vi "Gerador_de_Sinais.vi"() -> ()   [LabVIEW 2019]
uses:
  enum.ctl
  <vilib>/Utility/sysdir.llb/System Directory Type.ctl
  <vilib>/DAQmx/write.llb/DAQmx Write (Analog Wfm 1Chan NSamp).vi
  <vilib>/Waveform/WDTFileIO.llb/ Write Waveform to File.vi
  <vilib>/Waveform/WDTFileIO.llb/Read Waveform from File.vi
  <vilib>/Waveform/WDTOps.llb/WDT Append Waveforms DBL.vi
  <vilib>/DAQmx/create/channels.llb/DAQmx Create Channel (AO-Voltage-Basic).vi
  <vilib>/DAQmx/configure/timing.llb/DAQmx Timing (Use Waveform).vi
  <vilib>/DAQmx/miscellaneous.llb/DAQmx Fill In Error Info.vi
  <vilib>/measure/NI_MABase.lvlib
panel:
  in  "Nº de amostras":i32
  in  "Amostras/s":dbl
  in  "Canal out":tag
  in  "Input":tag
  in  "Adquirir":bool
  in  "Gerar":bool
  in  "Out mode":bool
  in  "Start":bool
  in  "conc-ops":bool
  in  "Ch2":bool
  in  "Ch1":bool
  in  "delete":bool
  in  "Escala X":dbl(knob)=0.5 min=0.5 step=0.5 scale=0.0..100.0
  in  "Conc":bool
  in  "Salvar 2":path
  in  "Salvar - opções 2":enum16{"Default", "Custom"}(ring)
  in  "Save 2":bool
  in  "Sub":bool
  in  "Add":bool
  in  "load2":bool
  in  "Carregar2":path
  out "Sinal 2":waveform(dbl)[](graph)
  in  "Salvar - opções":enum16{"Default", "Custom"}(ring)
  in  "Carregar1":path
  in  "Salvar":path
  in  "load1":bool
  in  "Save":bool
  in  "Parâmetros":T1={"Forma"=enum."Quadrada", "Amostragem"={"Amostras/s"=1000.0, "Qtde. de amostras"=1000.0}, "Frequência (Hz)"=1.0, "Amplitude (Vp)"=10.0, "Fase"=0.0, "Offset (V)"=0.0, "duty cycle (%)"=50.0} {"duty cycle (%)" format="%0.2f"; "Offset (V)" min=-10.0 max=10.0; "Fase" format="%.2p"; "Amplitude (Vp)" min=0.0 max=10.0 format="%#_13g"; "Frequência (Hz)" min=0.0 step=1.0; "Amostragem"."Qtde. de amostras" min=1000.0 step=1000.0; "Amostragem"."Amostras/s" min=0.0 format="%.2p"}
  out "Sinal":waveform(dbl)(graph)
  in  "stop":bool
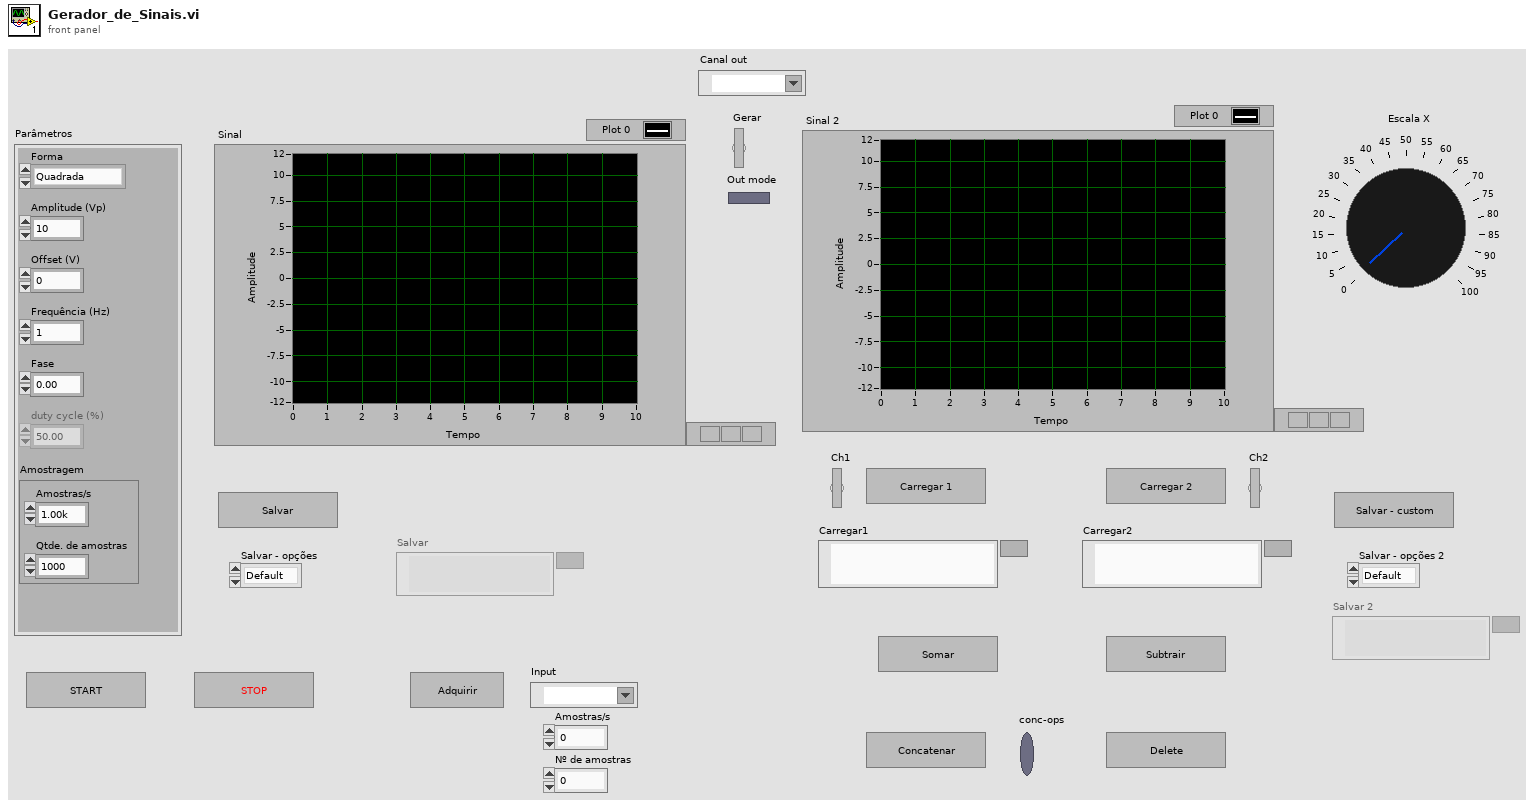
[diagram p1: front panel]
types:
  T1 = cluster{"Forma":enum16{"Quadrada", "Senoidal", "Triangular", "Dente de Serra", "Trapezoidal"}, "Amostragem":cluster{"Amostras/s":dbl, "Qtde. de amostras":dbl}, "Frequência (Hz)":dbl, "Amplitude (Vp)":dbl, "Fase":dbl, "Offset (V)":dbl, "duty cycle (%)":dbl}
  T2 = typedef "enum.ctl" = enum16{"update", "write", "stop", "save", "load1", "load2", "add", "sub", "delete", "display", "display -edit", "conc", "HW in", "HW out start", "HW out stop", "initialize", "canal out", "canal in", "save - custom"}
  T3 = cluster{"start":bool, "fila":cluster{"Operação":T2, "data":variant}}
  T4 = cluster{"onda1":waveform(dbl), "zero":waveform(dbl), "ch1":bool, "ch2":bool, "Parâmetros ":cluster{"Forma":enum16{"Quadrada", "Senoidal", "Triangular", "Dente de Serra", "Trapezoidal"}, "Amostragem":cluster{"Amostras/s":dbl, "Qtde. de amostras":dbl}, "Frequência (Hz)":dbl, "Amplitude (Vp)":dbl, "Fase":dbl, "Offset (V)":dbl, "duty cycle (%)":dbl}, "sinal":waveform(dbl), "stop ":bool, "Task out":refnum<k21>, "sinal in":waveform(dbl), "out":bool, "in":bool, "Canal in":tag, "onda 2":waveform(dbl)}
  T5 = enum8{"Enabled", "Disabled", "Disabled and Grayed Out"}
  T6 = enum16{"Quadrada", "Senoidal", "Triangular", "Dente de Serra", "Trapezoidal"}
  T7 = cluster{"Amostras/s":dbl, "Qtde. de amostras":dbl}
  T8 = typedef "System Directory Type.ctl" = i32
  T9 = typedef "LVCursorListTypeDef.ctl" = cluster{"Name":string, "Color":u32, "Style":u8, "Point Style":u8, "Name Visible":bool, "Allow Drag":bool, "Cursor Mode":u32, "Plot":i32, "Index":i32, "Position":cluster{"X":dbl, "Y":dbl}, "X Scale":u32, "Y Scale":u32, "Watch Plots":i32[], "Watch All Plots":bool, "Plot Area":i32, "Label Offset":cluster{"X":dbl, "Y":dbl}}[]
  T10 = cluster{"Name":string, "Color":u32, "Style":u8, "Point Style":u8, "Name Visible":bool, "Allow Drag":bool, "Cursor Mode":u32, "Plot":i32, "Index":i32, "Position":cluster{"X":dbl, "Y":dbl}, "X Scale":u32, "Y Scale":u32, "Watch Plots":i32[], "Watch All Plots":bool, "Plot Area":i32, "Label Offset":cluster{"X":dbl, "Y":dbl}}
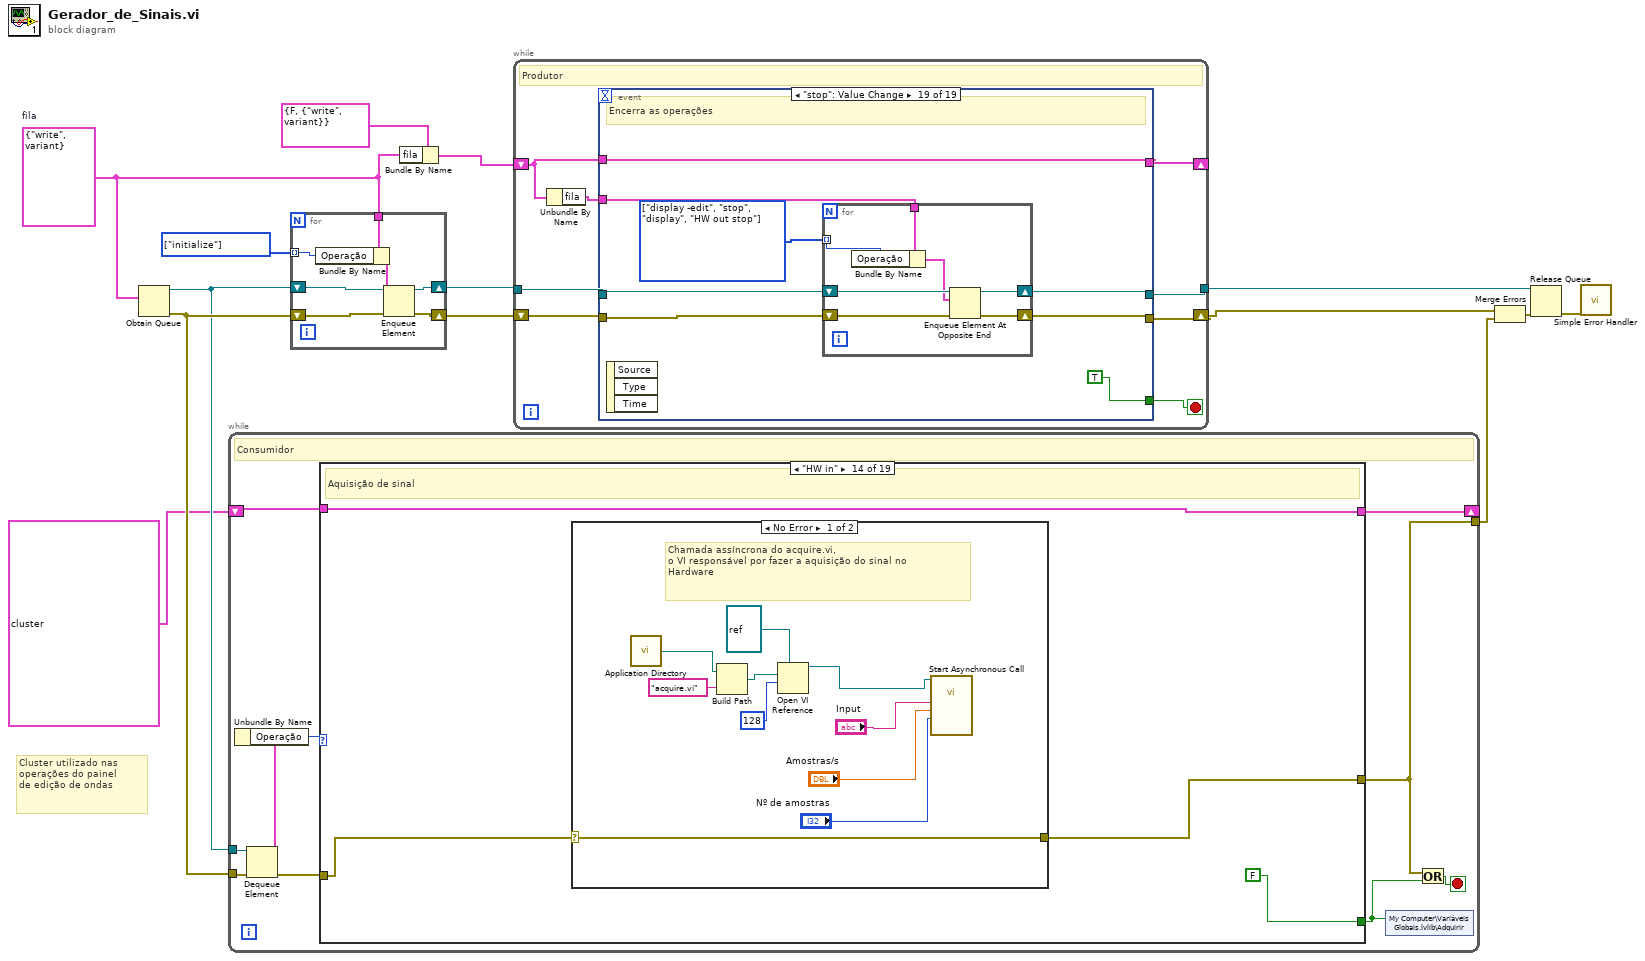
[diagram p0: block diagram]
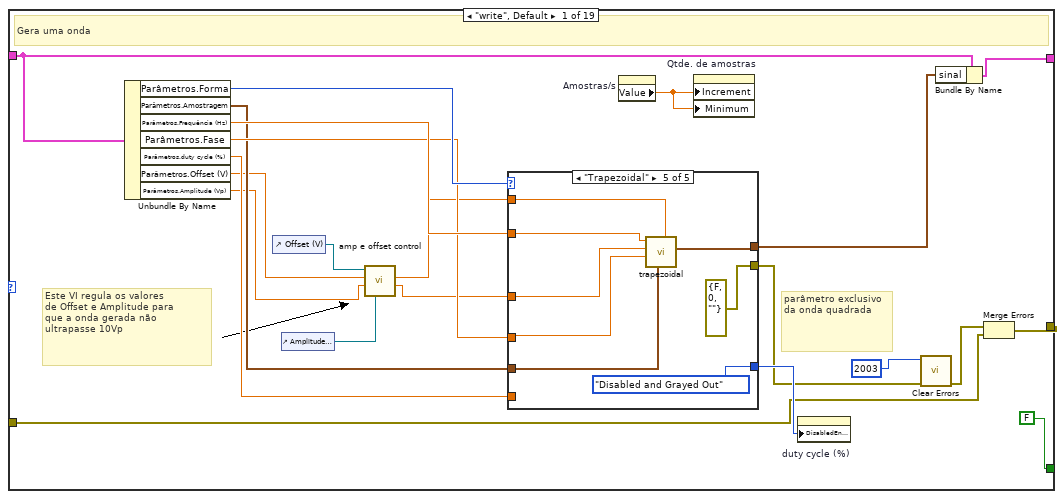
[diagram p2: hidden frame]
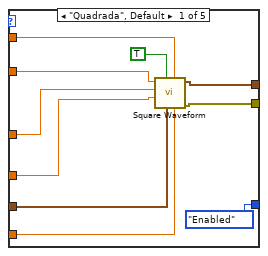
[diagram p3: hidden frame]
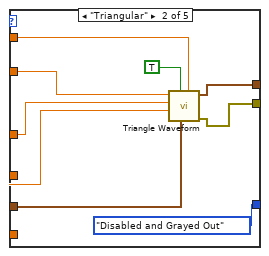
[diagram p4: hidden frame]
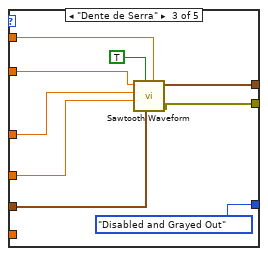
[diagram p5: hidden frame]
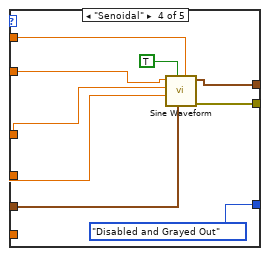
[diagram p6: hidden frame]
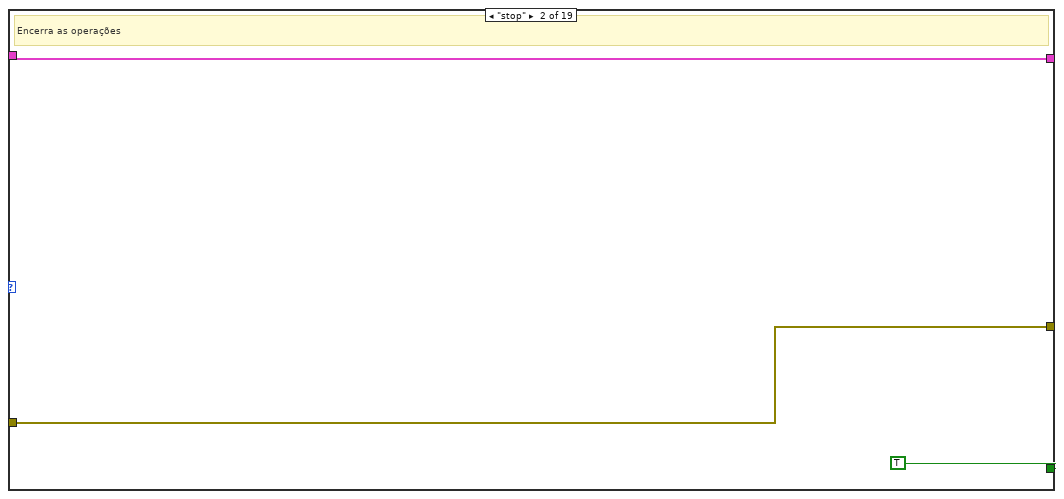
[diagram p7: hidden frame]
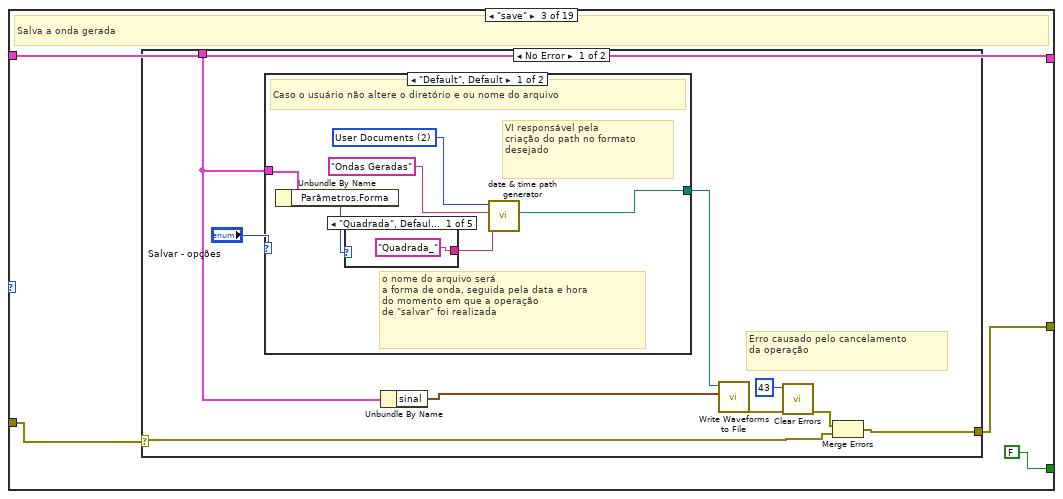
[diagram p8: hidden frame]
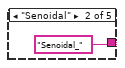
[diagram p9: hidden frame]
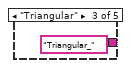
[diagram p10: hidden frame]
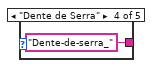
[diagram p11: hidden frame]
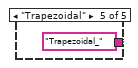
[diagram p12: hidden frame]
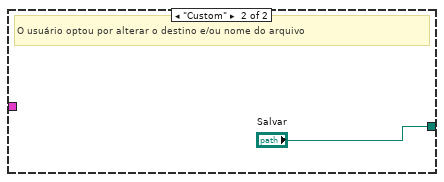
[diagram p13: hidden frame]
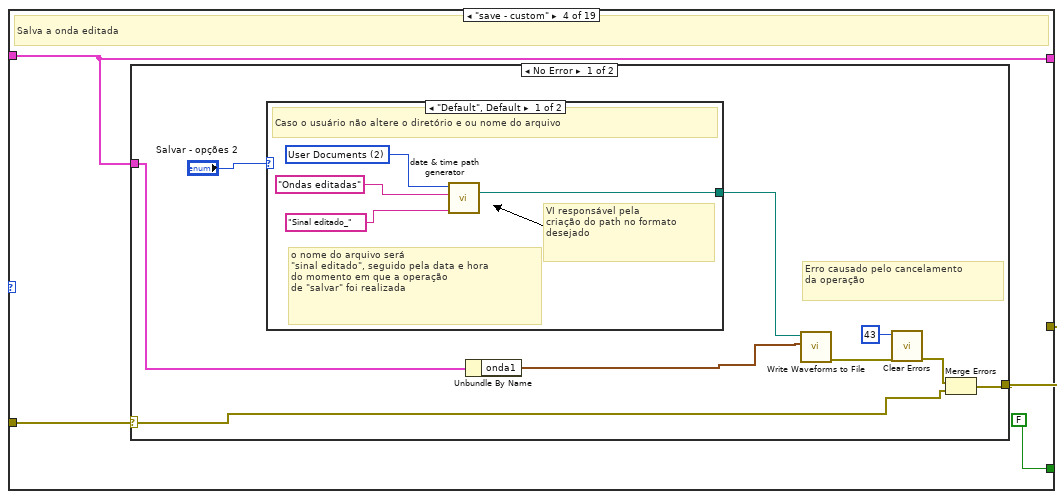
[diagram p15: hidden frame]
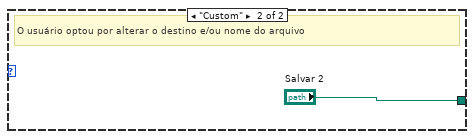
[diagram p16: hidden frame]
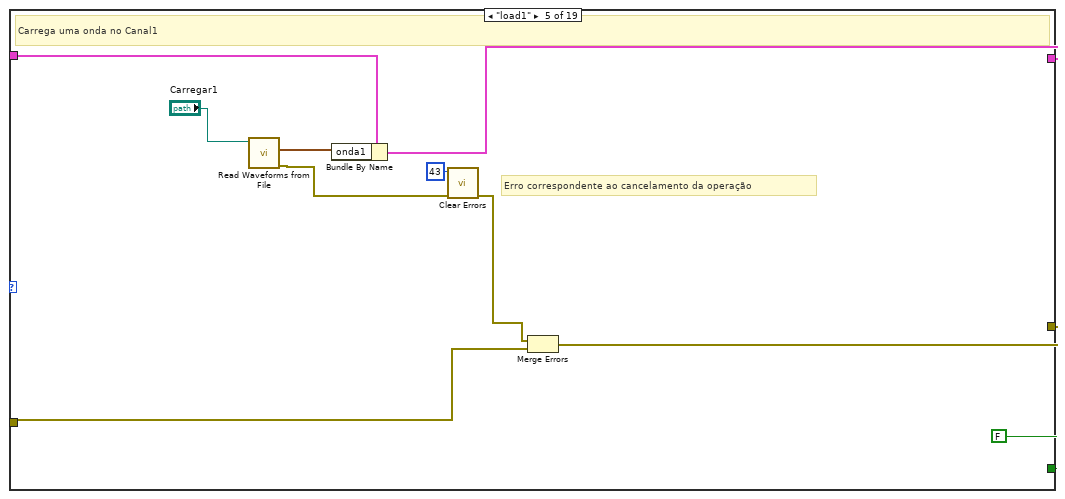
[diagram p18: hidden frame]
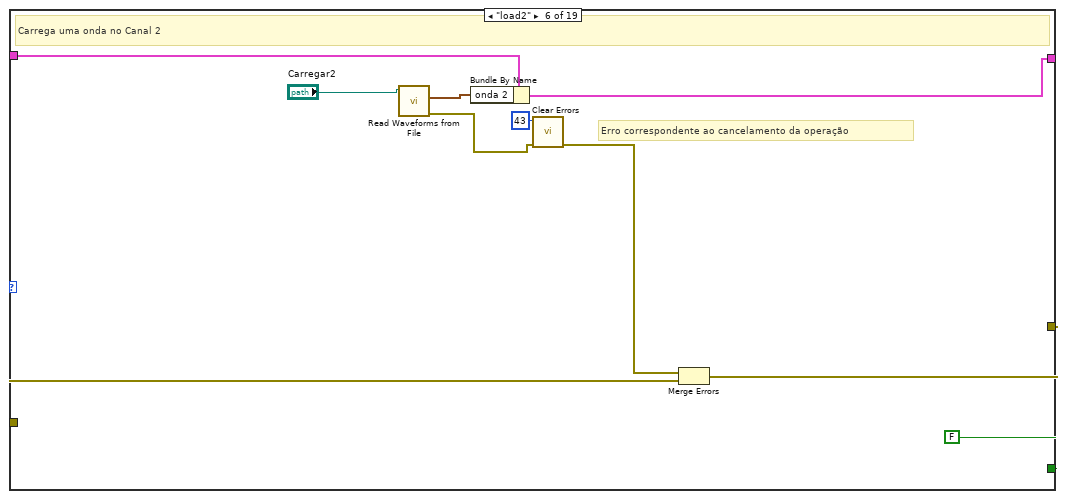
[diagram p19: hidden frame]
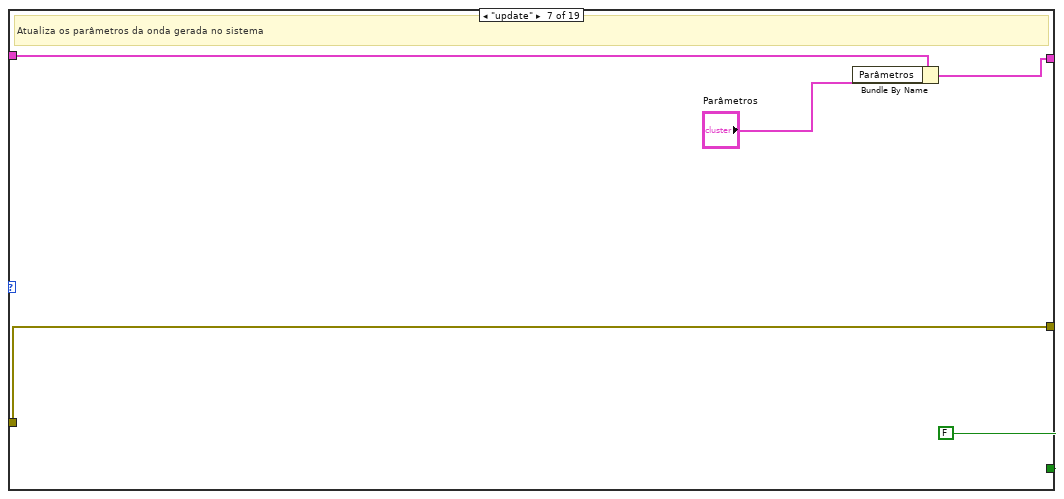
[diagram p20: hidden frame]
diagram:
  w5 = T2[] [enum."initialize"] items=["update", "write", "stop", "save", "load1", "load2", "add", "sub", "delete", "display", "display -edit", "conc", "HW in", "HW out start", "HW out stop", "initialize", "canal out", "canal in", "save - custom"]
  w4 = cluster{"Operação":T2, "data":variant} {"Operação"=enum."write", "data"=variant}  # fila
  # "Cluster utilizado nas \noperações do painel\nde edição de ondas"
  n1 = Obtain Queue(element data type=w4) -> (queue out=w11:refnum<queue>, error out=w12:errorcluster)  [unwired: 4 in, 1 out]
  n2 = while {
    shift-right: [w22] -> _
    shift-left: T4 {"onda1"={"t0"=timestamp(0 s since 1904-01-01), "dt"=1.0, "Y"=[]}, "zero"={"t0"=timestamp(0 s since 1904-01-01), "dt"=1.0, "Y"=[]}, "ch1"=TRUE, "ch2"=TRUE, "Parâmetros "={"Forma"=enum."Quadrada", "Amostragem"={"Amostras/s"=1000.0, "Qtde. de amostras"=1000.0}, "Frequência (Hz)"=1.0, "Amplitude (Vp)"=10.0, "Fase"=0.0, "Offset (V)"=0.0, "duty cycle (%)"=50.0}, "sinal"={"t0"=timestamp(0 s since 1904-01-01), "dt"=1.0, "Y"=[]}, "stop "=FALSE, "Task out"="", "sinal in"={"t0"=timestamp(0 s since 1904-01-01), "dt"=1.0, "Y"=[]}, "out"=FALSE, "in"=FALSE, "Canal in"="", "onda 2"={"t0"=timestamp(0 s since 1904-01-01), "dt"=1.0, "Y"=[]}} -> [w21]
    tunnel: w11 -> [w20]
    tunnel: w12 -> [w19]
    tunnel: [w17] -> w1
    stop <- w18 stop-if-true
    # "Consumidor"
    n3 = Dequeue Element(queue=w20, error in (no error)=w19) -> (element=w24:cluster{"Operação":T2, "data":variant}, error out=w16:errorcluster)  [unwired: 1 in, 2 out]
    n4 = Unbundle By Name(w24) -> ("Operação"=w23:T2)
    n5 = case shown="\"HW in\"" w23 {
      tunnel: [FALSE TRUE FALSE FALSE FALSE FALSE FALSE FALSE FALSE FALSE FALSE FALSE FALSE FALSE FALSE FALSE FALSE FALSE FALSE] -> w15
      tunnel: [w35 w94 w97 w123 w143 w153 w161 w173 w183 w189 w202 w226 w244 w255 w269 w302 w326 w335 w338] -> w22
      tunnel: w21 -> [w36 w94 w97 w123 w144 w154 w163 w172 w182 w188 w203 w225 w244 w255 w270 w302 w327 w336 w339]
      tunnel: w16 -> [w31 w93 w96 w121 w141 w151 w160 w165 w175 w186 w201 w223 w245 w254 w272 w300 w330 w332 w344]
      tunnel: [w33 w93 w95 w122 w140 w150 w160 w165 w175 w185 w201 w223 w245 w253 w271 w293 w329 w332 w343] -> w17
      frame "write", Default {
        # "Este VI regula os valores\nde Offset e Amplitude para\nque a onda gerada não\nultrapasse 10Vp"
        # "parâmetro exclusivo da onda quadrada"
        # "Gera uma onda"
        n6 = Unbundle By Name(w36) -> ("Parâmetros.Forma"=w43:T6, "Parâmetros.Amostragem"=w40:T7, "Parâmetros.Frequência (Hz)"=w44:dbl, "Parâmetros.Fase"=w42:dbl, "Parâmetros.duty cycle (%)"=w41:dbl, "Parâmetros.Offset (V)"=w26:dbl, "Parâmetros.Amplitude (Vp)"=w25:dbl)
        n7 = control-ref of="Offset (V)"() -> (w30:refnum<vi>)
        n8 = control-ref of="Amplitude (Vp)"() -> (w29:refnum<vi>)
        n9 = call "amp e offset control.vi"("amp ref"=w29, "Amplitude (Vp)"=w25, "Offset (V)"=w26, "offset ref"=w30) -> ("Nova Amplitude"=w28:dbl, "Novo Offset"=w27:dbl)  [unwired: 6 in]
        n10 = case shown="\"Trapezoidal\"" w43 {
          tunnel: [w56 w65 w74 w83 w90] -> w34
          tunnel: w28 -> [w55 w64 w73 w82 w91]
          tunnel: [T5."Enabled" ("Disabled") T5."Disabled and Grayed Out" ("Disabled") T5."Disabled and Grayed Out" ("Disabled") T5."Disabled and Grayed Out" ("Disabled") T5."Disabled and Grayed Out" ("Disabled")] -> w45
          tunnel: w27 -> [w51 w60 w69 w79 w87]
          tunnel: w44 -> [w52 w61 w70 w78 w88]
          tunnel: w42 -> [w50 w59 w68 w77 w86]
          tunnel: w41 -> [w49 _ _ _ _]
          tunnel: w40 -> [w48 w58 w67 w76 w85]
          tunnel: [w47 w57 w66 w75 errorcluster {"status"=FALSE, "code"=0, "source"=""} ("error out")] -> w39
          frame "Quadrada", Default {
            n11 = call <vilib>:"Square Waveform.vi"("duty cycle (%)"=w49, "offset"=w51, "sampling info"=w48, "reset signal"=TRUE, "phase"=w50, "amplitude"=w55, "frequency"=w52) -> ("error out"=w47:errorcluster, "signal out"=w56:waveform(dbl))  [unwired: 3 in]
          }
          frame "Triangular" {
            n12 = call <vilib>:"Triangle Waveform.vi"("offset"=w60, "sampling info"=w58, "reset signal"=TRUE, "phase"=w59, "amplitude"=w64, "frequency"=w61) -> ("error out"=w57:errorcluster, "signal out"=w65:waveform(dbl))  [unwired: 4 in]
          }
          frame "Dente de Serra" {
            n13 = call <vilib>:"Sawtooth Waveform.vi"("offset"=w69, "sampling info"=w67, "reset signal"=TRUE, "phase"=w68, "amplitude"=w73, "frequency"=w70) -> ("error out"=w66:errorcluster, "signal out"=w74:waveform(dbl))  [unwired: 4 in]
          }
          frame "Senoidal" {
            n14 = call <vilib>:"Sine Waveform.vi"("offset"=w79, "sampling info"=w76, "reset signal"=TRUE, "phase"=w77, "amplitude"=w82, "frequency"=w78) -> ("error out"=w75:errorcluster, "signal out"=w83:waveform(dbl))  [unwired: 4 in]
          }
          frame "Trapezoidal" {
            n15 = call "trapezoidal.vi"("offset"=w87, "sampling info"=w85, "phase"=w86, "amplitude"=w91, "frequency"=w88) -> ("signal"=w90:waveform(dbl))  [unwired: 6 in]
          }
        }
        n16 = property on="Amostras/s" class="DigNum (strict)"() -> ("Value"=w37:dbl)  [unwired: 2 in, 2 out]
        n17 = property on="Qtde. de amostras" class="DigNum (strict)"("Increment"=w37, "Minimum"=w37) -> ()  [unwired: 2 in, 2 out]
        n18 = property on="duty cycle (%)" class="DigNum (strict)"("DisabledEnum"=w45) -> ()  [unwired: 2 in, 2 out]
        n19 = call <vilib>:"Clear Errors.vi"("error in (no error)"=w39, "specific error code to clear (0: all)"=2003) -> ("error out"=w32:errorcluster)  [unwired: 4 in, 1 out]
        n20 = Bundle By Name(cluster=w36, "sinal"=w34) -> (w35:T4)
        n21 = Merge Errors(w32, w31) -> (w33:errorcluster)
      }
      frame "stop" {
        # "Encerra as operações"
      }
      frame "save" {
        # "Salva a onda gerada"
        n22 = case shown="No Error" w96 {
          selector: w96 -> [w99 w120]
          tunnel: w97 -> [w103 _]
          tunnel: [w100 w120] -> w95
          frame No Error {
            # "Erro causado pelo cancelamento\nda operação"
            n23 = case shown="\"Default\", Default" "Salvar - opções" {
              tunnel: w103 -> [w112 _]
              tunnel: [w111 "Salvar"] -> w104
              frame "Default", Default {
                w108 = T8 2 items=["User Home"=0, "User Desktop"=1, "User Documents"=2, "User Application Data"=3, "User Preferences"=4, "User Temporary"=5, "Public Documents"=6, "Public Application Data"=7, "Public Preferences"=8, "Public Cache"=13, "System Core Libraries"=9, "System Installed Libraries"=10, "Application Files"=11, "Boot Volume Root"=12] ("system directory type")
                # "VI responsável pela\ncriação do path no formato\ndesejado"
                # "o nome do arquivo será \na forma de onda, seguida pela data e hora \ndo momento em que a operação\nde \"salvar\" foi realizada"
                # "Caso o usuário não altere o diretório e ou nome do arquivo"
                n24 = Unbundle By Name(w112) -> ("Parâmetros.Forma"=w113:T6)
                n25 = case shown="\"Quadrada\", Default" w113 {
                  tunnel: ["Quadrada_" "Senoidal_" "Triangular_" "Dente-de-serra_" "Trapezoidal_"] -> w109
                  frame "Quadrada", Default {
                  }
                  frame "Senoidal" {
                  }
                  frame "Triangular" {
                  }
                  frame "Dente de Serra" {
                  }
                  frame "Trapezoidal" {
                  }
                }
                n26 = call "date & time path generator.vi"("system directory type"=w108, "nome da pasta"="Ondas Geradas" ("prompt (Create Folder)"), "nome do arquivo"=w109) -> ("path"=w111:path)  [unwired: 7 in]
              }
              frame "Custom" {
                # "O usuário optou por alterar o destino e/ou nome do arquivo"
              }
            }
            n27 = Unbundle By Name(w103) -> ("sinal"=w102:waveform(dbl))
            n28 = call-poly <vilib>:"Write Waveforms to File.vi"("waveform"=w102, "file path (dialog if empty)"=w104) -> ("error out"=w106:errorcluster)  [unwired: 8 in, 1 out]
            n29 = call <vilib>:"Clear Errors.vi"("error in (no error)"=w106, "specific error code to clear (0: all)"=43) -> ("error out"=w101:errorcluster)  [unwired: 4 in, 1 out]
            n30 = Merge Errors(w101, w99) -> (w100:errorcluster)
          }
          frame Error {
          }
        }
      }
      frame "save - custom" {
        # "Salva a onda editada"
        n31 = case shown="No Error" w121 {
          selector: w121 -> [w125 w139]
          tunnel: w123 -> [w128 _]
          tunnel: [w126 w139] -> w122
          frame No Error {
            # "Erro causado pelo cancelamento\nda operação"
            n32 = case shown="\"Default\", Default" "Salvar - opções 2" {
              tunnel: [w137 "Salvar 2"] -> w132
              frame "Default", Default {
                w136 = T8 2 items=["User Home"=0, "User Desktop"=1, "User Documents"=2, "User Application Data"=3, "User Preferences"=4, "User Temporary"=5, "Public Documents"=6, "Public Application Data"=7, "Public Preferences"=8, "Public Cache"=13, "System Core Libraries"=9, "System Installed Libraries"=10, "Application Files"=11, "Boot Volume Root"=12] ("system directory type")
                # "VI responsável pela\ncriação do path no formato\ndesejado"
                # "o nome do arquivo será \n\"sinal editado\", seguido pela data e hora \ndo momento em que a operação\nde \"salvar\" foi realizada"
                # "Caso o usuário não altere o diretório e ou nome do arquivo"
                n33 = call "date & time path generator.vi"("system directory type"=w136, "nome da pasta"="Ondas editadas" ("prompt (Create Folder)"), "nome do arquivo"="Sinal editado_") -> ("path"=w137:path)  [unwired: 7 in]
              }
              frame "Custom" {
                # "O usuário optou por alterar o destino e/ou nome do arquivo"
              }
            }
            n34 = Unbundle By Name(w128) -> ("onda1"=w131:waveform(dbl))
            n35 = call-poly <vilib>:"Write Waveforms to File.vi"("waveform"=w131, "file path (dialog if empty)"=w132) -> ("error out"=w130:errorcluster)  [unwired: 8 in, 1 out]
            n36 = call <vilib>:"Clear Errors.vi"("error in (no error)"=w130, "specific error code to clear (0: all)"=43) -> ("error out"=w127:errorcluster)  [unwired: 4 in, 1 out]
            n37 = Merge Errors(w127, w125) -> (w126:errorcluster)
          }
          frame Error {
          }
        }
      }
      frame "load1" {
        # "Erro correspondente ao cancelamento da operação"
        # "Carrega uma onda no Canal1"
        n38 = call-poly <vilib>:"Read Waveforms from File.vi"("file path (dialog if empty)"="Carregar1") -> ("error out"=w145:errorcluster, "first waveform in record"=w147:waveform(dbl))  [unwired: 5 in, 2 out]
        n39 = Bundle By Name(cluster=w144, "onda1"=w147) -> (w143:T4)
        n40 = call <vilib>:"Clear Errors.vi"("error in (no error)"=w145, "specific error code to clear (0: all)"=43) -> ("error out"=w142:errorcluster)  [unwired: 4 in, 1 out]
        n41 = Merge Errors(w142, w141) -> (w140:errorcluster)
      }
      frame "load2" {
        # "Erro correspondente ao cancelamento da operação"
        # "Carrega uma onda no Canal 2"
        n42 = call-poly <vilib>:"Read Waveforms from File.vi"("file path (dialog if empty)"="Carregar2") -> ("error out"=w156:errorcluster, "first waveform in record"=w157:waveform(dbl))  [unwired: 5 in, 2 out]
        n43 = Bundle By Name(cluster=w154, "onda 2"=w157) -> (w153:T4)
        n44 = call <vilib>:"Clear Errors.vi"("error in (no error)"=w156, "specific error code to clear (0: all)"=43) -> ("error out"=w152:errorcluster)  [unwired: 4 in, 1 out]
        n45 = Merge Errors(w152, w151) -> (w150:errorcluster)
      }
      frame "update" {
        # "Atualiza os parâmetros da onda gerada no sistema"
        n46 = Bundle By Name(cluster=w163, "Parâmetros"="Parâmetros") -> (w161:T4)
      }
      frame "add" {
        # "o sinal resultante substitui aquele carregado no canal1"
        # "adição dos sinais do canal 1 e do \ncanal2 e normalização do sinal resultante \ndentro do limite estabelicdo"
        # "Adição de 2 ondas"
        n47 = Unbundle By Name(w172) -> ("onda1"=w167:waveform(dbl), "onda 2"=w166:waveform(dbl))
        n48 = call "add or sub waveforms.vi"("operation"=TRUE, "inf"=-10.0, "Waveform 2"=w166, "Waveform 1"=w167, "sup"=10.0) -> ("New Waveform"=w168:waveform(dbl))  [unwired: 6 in]
        n49 = Bundle By Name(cluster=w172, "onda1"=w168) -> (w173:T4)
      }
      frame "sub" {
        # "subtração dos sinais do canal 1 e do \ncanal2 e normalização do sinal resultante \ndentro do limite estabelicdo"
        # "o sinal resultante substitui aquele carregado no canal1"
        # "Subtração de 2 ondas"
        n50 = Unbundle By Name(w182) -> ("onda1"=w181:waveform(dbl), "onda 2"=w180:waveform(dbl))
        n51 = call "add or sub waveforms.vi"("operation"=FALSE, "inf"=-10.0, "Waveform 2"=w180, "Waveform 1"=w181, "sup"=10.0) -> ("New Waveform"=w179:waveform(dbl))  [unwired: 6 in]
        n52 = Bundle By Name(cluster=w182, "onda1"=w179) -> (w183:T4)
      }
      frame "conc" {
        # "Concatenar 2 ondas"
        n53 = Unbundle By Name(w188) -> ("onda1"=w194:waveform(dbl), "onda 2"=w192:waveform(dbl))
        n54 = case shown="True" "conc-ops" {
          tunnel: [w198 w199] -> w193
          tunnel: w194 -> [w198 w200]
          tunnel: w192 -> [w197 w199]
          tunnel: [w197 w200] -> w191
          frame False {
            # "A onda2 começa depois da1"
          }
          frame True {
            # "A onda 2 começa antes da 1"
          }
        }
        n55 = call-poly <vilib>:"Append Waveforms.vi"("waveform B"=w191, "waveform A"=w193) -> ("error out"=w187:errorcluster, "waveform out"=w195:waveform(dbl))  [unwired: 8 in]
        n56 = Bundle By Name(cluster=w188, "onda1"=w195) -> (w189:T4)
        n57 = Merge Errors(w187, w186) -> (w185:errorcluster)
      }
      frame "delete" {
        # "Deleta o trecho \"entre cursores\"da onda apresentada no display"
        n58 = Unbundle By Name(w203) -> ("ch1"=w204:bool, "ch2"=w205:bool)
        n59 = Or(x=w204, y=w205) -> (x .or. y?=w206:bool)
        n60 = case shown="True" w206 {
          tunnel: w203 -> [w208 w213]
          tunnel: [w208 w216] -> w202
          tunnel: w204 -> [_ w212]
          frame False {
            # "Se os dois canais estiverem desabilitados, nada acontece"
          }
          frame True {
            # "Se o canal1 estiver\nativo, sua onda será editada.\nCaso o contrário, a onda do canal2 será \neditada"
            # "Pelo menos um canal está ativo"
            n61 = Unbundle By Name(w213) -> ("onda1"=w215:waveform(dbl), "onda 2"=w214:waveform(dbl))
            n62 = Select(t=w215, s=w212, f=w214) -> (s? t:f=w211:waveform(dbl))
            n63 = control-ref of="Sinal 2"() -> (w209:refnum<vi>)
            n64 = call "deleta trecho de onda.vi"("Waveform"=w211, "reference"=w209) -> ("New Waveform"=w210:waveform(dbl))  [unwired: 9 in]
            n65 = case shown="True" w212 {
              tunnel: w210 -> [w219 w222]
              tunnel: [w217 w221] -> w216
              tunnel: w213 -> [w218 w220]
              frame False {
                # "A onda 2 foi editada"
                n66 = Bundle By Name(cluster=w218, "onda 2"=w219) -> (w217:T4)
              }
              frame True {
                # "A onda1 foi editada"
                n67 = Bundle By Name(cluster=w220, "onda1"=w222) -> (w221:T4)
              }
            }
          }
        }
      }
      frame "display -edit" {
        # "Atualiza o display de edição"
        n68 = Bundle By Name(cluster=w225, "ch2"="Ch2", "ch1"="Ch1", "stop"="stop") -> (w230:T4)
        n69 = case shown="True" "stop" {
          tunnel: w230 -> [w240 w243]
          tunnel: [w240 w243] -> w226
          tunnel: "Ch1" -> [w239 _]
          tunnel: "Ch2" -> [w237 _]
          tunnel: [w238 w242] -> w227
          frame False {
            # "canal 1"
            # "canal 2"
            # "Stop não foi pressionado"
            n70 = Unbundle By Name(w240) -> ("onda 2"=w235:waveform(dbl), "zero"=w234:waveform(dbl), "onda1"=w236:waveform(dbl))
            n71 = Select(t=w235, s=w237, f=w234) -> (s? t:f=w232:waveform(dbl))
            n72 = Select(t=w236, s=w239, f=w234) -> (s? t:f=w233:waveform(dbl))
            n73 = Build Array(w233, w232) -> (w238:waveform(dbl)[])
          }
          frame True {
            # "Limpa o display"
            # "Stop foi pressionado"
            n74 = Unbundle By Name(w243) -> ("zero"=w241:waveform(dbl))
            n75 = Build Array(w241, w241) -> (w242:waveform(dbl)[])
          }
        }
        "Sinal 2" <- w227
      }
      frame "display" {
        n76 = Unbundle By Name(w244) -> ("stop"=w248:bool)
        n77 = case shown="True" w248 {
          tunnel: w244 -> [w250 w252]
          tunnel: [w249 w251] -> w247
          frame False {
            n78 = Unbundle By Name(w250) -> ("sinal"=w249:waveform(dbl))
          }
          frame True {
            n79 = Unbundle By Name(w252) -> ("zero"=w251:waveform(dbl))
          }
        }
        "Sinal" <- w247
      }
      frame "HW in" {
        # "Aquisição de sinal"
        n80 = case shown="No Error" w254 {
          selector: w254 -> [w257 w267]
          tunnel: [w257 w267] -> w253
          frame No Error {
            # "Chamada assíncrona do acquire.vi,\no VI responsável por fazer a aquisição do sinal no\nHardware"
            n81 = call <vilib>:"Application Directory.vi"() -> ("Application Directory"=w266:path)
            n82 = Build Path(base path=w266, name or relative path="acquire.vi") -> (appended path=w264:path)
            n83 = Open VI Reference(type specifier VI Refnum (for type only)=refnum<vi> refnum, vi path=w264, options=128) -> (vi reference=w262:refnum<vi>)  [unwired: 3 in, 1 out]
            n84 = call-by-ref "Start Asynchronous Call"(reference=w262, "Number of Samples"="Nº de amostras", "Sample Rate"="Amostras/s", "Physical Channel"="Input") -> ()  [unwired: 9 in, 3 out]
          }
          frame Error {
          }
        }
      }
      frame "HW out start" {
        # "Gerar forma de onda no HW"
        n85 = case shown="No Error" w272 {
          selector: w272 -> [w289 w291]
          tunnel: w270 -> [w274 w292]
          tunnel: [w287 w291] -> w271
          tunnel: [w290 w292] -> w269
          frame No Error {
            w283 = 10123 items=["Finite Samples"=10178, "Continuous Samples"=10123, "Hardware Timed Single Point"=12522] ("sample mode")
            # "Flag \"out\" será utilizada \nno estado HW out stop, \npara que o programa verifique\nse é necessário finalizar a task antes\nde encerrar o VI"
            # "seleciona a onda a ser\ngerada no HW."
            n86 = Unbundle By Name(w274) -> ("onda1"=w285:waveform(dbl), "sinal"=w284:waveform(dbl))
            n87 = call-poly <vilib>:"DAQmx Create Virtual Channel.vi"("physical channels"="Canal out", "error in"=w289) -> ("task out"=w276:refnum<k21>, "error out"=w277:errorcluster)  [unwired: 12 in]
            n88 = Select(t=w285, s="Out mode", f=w284) -> (s? t:f=w282:waveform(dbl))
            n89 = call-poly <vilib>:"DAQmx Timing.vi"("task/channels in"=w276, "sample mode"=w283, "waveform"=w282, "error in"=w277) -> ("task out"=w281:refnum<k21>, "error out"=w280:errorcluster)  [unwired: 10 in]
            n90 = call-poly <vilib>:"DAQmx Write.vi"("task/channels in"=w281, "data"=w282, "error in"=w280) -> ("task out"=w279:refnum<k21>, "error out"=w278:errorcluster)  [unwired: 10 in, 1 out]
            n91 = call <vilib>:"DAQmx Start Task.vi"("task/channels in"=w279, "error in"=w278) -> ("task out"=w288:refnum<k21>, "error out"=w287:errorcluster)  [unwired: 12 in]
            n92 = Bundle By Name(cluster=w274, "Task out"=w288, "out"=TRUE) -> (w290:T4)
          }
          frame Error {
          }
        }
      }
      frame "initialize" {
        w296 = T5."Enabled" ("Disabled")
        w303 = 1000.0 ("Value")
        # "Inicialização do programa"
        n93 = property on="Sinal 2" class="WFGraph (strict)"(error in=w300) -> (error out=w299:errorcluster, "CrsrList"=w317:T9)  [unwired: 1 in, 1 out]
        n94 = Index Array(array=w317, index=1) -> (element=w316:T10)
        n95 = Index Array(array=w317, index=0) -> (element=w315:T10)
        n96 = Bundle By Name(cluster=w316, "Position.Y"=0.0) -> (w319:T10)
        n97 = property on="Adquirir" class="Bool"(error in=w299, "DisabledEnum"=w296) -> (error out=w298:errorcluster)  [unwired: 1 in, 1 out]
        n98 = Bundle By Name(cluster=w315, "Position.Y"=0.0) -> (w318:T10)
        n99 = property on="Gerar" class="Bool (strict)"(error in=w298, "DisabledEnum"=w296) -> (error out=w297:errorcluster)  [unwired: 1 in, 1 out]
        n100 = Replace Array Subset(array=w317, new element=w318, index=0) -> (w320:T9)
        n101 = Replace Array Subset(array=w320, new element=w319, index=1) -> (w321:T9)
        n102 = property on="Sinal 2" class="WFGraph (strict)"(error in=w297, "CrsrList"=w321) -> (error out=w322:errorcluster)  [unwired: 1 in, 1 out]
        n103 = property on="Salvar - opções" class="Enum (strict)"(error in=w322, "Value"=enum16{"Default", "Custom"}."Default" ("Salvar - opções")) -> (error out=w314:errorcluster)  [unwired: 1 in, 1 out]
        n104 = property on="Salvar" class="Path"(error in=w314, "DisabledEnum"=T5."Disabled and Grayed Out" ("Disabled")) -> (error out=w312:errorcluster)  [unwired: 1 in, 1 out]
        n105 = property on="Amostras/s" class="DigNum (strict)"(error in=w312, "Value"=w303) -> (error out=w313:errorcluster)  [unwired: 1 in, 1 out]
        n106 = property on="Qtde. de amostras" class="DigNum (strict)"(error in=w313, "Value"=w303) -> (error out=w295:errorcluster)  [unwired: 1 in, 1 out]
        n107 = property on="Gerar" class="Bool (strict)"(error in=w295, "Value"=FALSE ("Gerar")) -> (error out=w293:errorcluster)  [unwired: 1 in, 1 out]
      }
      frame "canal out" {
        # "Seleção do canal de saída"
        n108 = property on="Gerar" class="Bool (strict)"("DisabledEnum"=T5."Enabled" ("Disabled")) -> ()  [unwired: 2 in, 2 out]
        n109 = call-poly <vilib>:"DAQmx Create Virtual Channel.vi"("physical channels"=tag "Dev1/ao0", "error in"=w330) -> ("task out"=w328:refnum<k21>, "error out"=w329:errorcluster)  [unwired: 12 in]
        n110 = Bundle By Name(cluster=w327, "Task out"=w328) -> (w326:T4)
      }
      frame "canal in" {
        w331 = tag ""  # Canal in
        n111 = property on="Adquirir" class="Bool"("DisabledEnum"=T5."Enabled" ("Disabled")) -> ()  [unwired: 2 in, 2 out]
        n112 = Bundle By Name(cluster=w336, "Canal in"=w331) -> (w335:T4)
      }
      frame "HW out stop" {
        # "A flag \"out\" indica se\né necessário interromper a task ao\nchegar neste estado"
        # "Finaliza a task do output do HW"
        n113 = Unbundle By Name(w339) -> ("out"=w340:bool, "Task out"=w341:refnum<k21>)
        n114 = case shown="False" w340 {
          tunnel: w344 -> [w345 w350]
          tunnel: [w345 w347] -> w343
          tunnel: w341 -> [_ w348]
          frame False {
          }
          frame True {
            n115 = call <vilib>:"DAQmx Stop Task.vi"("task/channels in"=w348, "error in"=w350) -> ("task out"=w346:refnum<k21>, "error out"=w349:errorcluster)  [unwired: 12 in]
            n116 = call <vilib>:"DAQmx Clear Task.vi"("task in"=w346, "error in"=w349) -> ("error out"=w347:errorcluster)  [unwired: 13 in]
          }
        }
        n117 = Bundle By Name(cluster=w339, "out"=FALSE) -> (w338:T4)
      }
    }
    n118 = shared-variable "My Computer\\Variáveis Globais.lvlib\\Adquirir"(w15) -> ()  [unwired: 1 in, 1 out]
    n119 = Or(x=w17, y=w15) -> (x .or. y?=w18:bool)
  }
  n120 = for {
    tunnel: w4 -> [w352]
    shift-right: [w353] -> w8
    shift-left: w12 -> [w357]
    shift-right: [w354] -> w9
    shift-left: w11 -> [w356]
    tunnel: w5 -> [w351] mode=indexing
    n121 = Bundle By Name(cluster=w352, "Operação"=w351) -> (w355:cluster{"Operação":T2, "data":variant})
    n122 = Enqueue Element(queue=w356, element=w355, error in (no error)=w357) -> (queue out=w354:refnum<queue>, error out=w353:errorcluster)  [unwired: 1 in, 1 out]
  }
  n123 = Bundle By Name(cluster=T3 {"start"=FALSE, "fila"={"Operação"=enum."write", "data"=variant}}, "fila"=w4) -> (w7:T3)
  n124 = while {
    shift-right: [w363] -> w2
    shift-left: w8 -> [w361]
    tunnel: w9 -> [w362]
    tunnel: [w364] -> w14
    shift-right: [w358] -> _
    shift-left: w7 -> [w360]
    stop <- w365 stop-if-true
    # "Produtor"
    n125 = Unbundle By Name(w360) -> ("fila"=w359:cluster{"Operação":T2, "data":variant})
    n126 = event shown="[18] \"stop\": Value Change" {
      selector: _ -> [_ _ _ _ _ _ _ _ _ _ _ _ _ _ _ _ _ _ _]
      dyn-events: _ -> [_ _ _ _ _ _ _ _ _ _ _ _ _ _ _ _ _ _ _]
      timeout: _ -> [_ _ _ _ _ _ _ _ _ _ _ _ _ _ _ _ _ _ _]
      tunnel: w362 -> [w372 w397 w409 w418 w432 w449 w461 w476 w491 w509 w520 w527 w542 w557 w569 w578 w587 w596 w606]
      tunnel: w361 -> [w371 w396 w410 w419 w430 w446 w462 w477 w492 w510 w518 w528 w543 w558 w568 w577 w586 w595 w605]
      tunnel: [FALSE FALSE FALSE FALSE FALSE FALSE FALSE FALSE FALSE FALSE FALSE FALSE FALSE FALSE FALSE FALSE FALSE FALSE TRUE] -> w365
      tunnel: [w370 w394 w411 w420 w427 w441 w459 w474 w489 w511 w517 w525 w540 w555 w568 w579 w588 w597 w603] -> w363
      tunnel: [w369 w395 w412 w421 w431 w448 w460 w475 w490 w512 w516 w526 w541 w556 w569 w580 w589 w598 w604] -> w364
      tunnel: [w367 w391 w407 w416 w424 w440 w458 w473 w488 w506 w519 w524 w539 w554 w567 w574 w583 w592 w602] -> w358
      tunnel: w360 -> [w367 w392 w407 w416 w424 w440 w458 w473 w488 w506 w519 w524 w539 w554 w567 w574 w583 w592 w602]
      tunnel: w359 -> [w366 w390 w406 w415 _ _ w457 w472 w487 w505 w515 w523 w538 w553 _ w573 w582 w591 w601]
      event "Parâmetros": Value Change {
        # "Se houver uma alteração em qualquer parâmetro do sinal, uma nova Waveform é gerada"
        n127 = event-data() -> ()  [unwired: 1 in, 3 out]
        n128 = Unbundle By Name(w367) -> ("start"=w368:bool)
        n129 = case shown="True" w368 {
          tunnel: w372 -> [w375 w381]
          tunnel: w371 -> [w374 w380]
          tunnel: [w374 w378] -> w370
          tunnel: [w375 w379] -> w369
          tunnel: w366 -> [_ w377]
          frame False {
          }
          frame True {
            w376 = T2[] [enum."update", enum."write", enum."display"] items=["update", "write", "stop", "save", "load1", "load2", "add", "sub", "delete", "display", "display -edit", "conc", "HW in", "HW out start", "HW out stop", "initialize", "canal out", "canal in", "save - custom"]
            n130 = for {
              tunnel: w377 -> [w384]
              tunnel: w376 -> [w382] mode=indexing
              shift-right: [w386] -> w379
              shift-left: w381 -> [w388]
              shift-right: [w385] -> w378
              shift-left: w380 -> [w387]
              n131 = Bundle By Name(cluster=w384, "Operação"=w382) -> (w383:cluster{"Operação":T2, "data":variant})
              n132 = Enqueue Element(queue=w388, element=w383, error in (no error)=w387) -> (queue out=w386:refnum<queue>, error out=w385:errorcluster)  [unwired: 1 in, 1 out]
            }
          }
        }
      }
      event "Start": Value Change {
        w389 = T2[] [enum."update", enum."write", enum."display"] items=["update", "write", "stop", "save", "load1", "load2", "add", "sub", "delete", "display", "display -edit", "conc", "HW in", "HW out start", "HW out stop", "initialize", "canal out", "canal in", "save - custom"]
        # "Se houver uma alteração em qualquer parâmetro do sinal, uma nova Waveform é gerada"
        n133 = event-data() -> ()  [unwired: 1 in, 5 out]
        n134 = for {
          tunnel: w389 -> [w399] mode=indexing
          tunnel: w390 -> [w400]
          shift-right: [w403] -> w395
          shift-left: w397 -> [w405]
          shift-right: [w402] -> w394
          shift-left: w396 -> [w404]
          n135 = Bundle By Name(cluster=w400, "Operação"=w399) -> (w401:cluster{"Operação":T2, "data":variant})
          n136 = Enqueue Element(queue=w405, element=w401, error in (no error)=w404) -> (queue out=w403:refnum<queue>, error out=w402:errorcluster)  [unwired: 1 in, 1 out]
        }
        n137 = Bundle By Name(cluster=w392, "start"="Start") -> (w391:T3)
      }
      event "Save": Value Change {
        # "Salvar a onda gerada"
        n138 = event-data() -> ()  [unwired: 1 in, 5 out]
        n139 = Bundle By Name(cluster=w406, "Operação"=enum."save") -> (w408:cluster{"Operação":T2, "data":variant})
        n140 = Enqueue Element(queue=w409, element=w408, error in (no error)=w410) -> (queue out=w412:refnum<queue>, error out=w411:errorcluster)  [unwired: 1 in, 1 out]
      }
      event "Save 2": Value Change {
        # "Salvar a onda editada"
        n141 = event-data() -> ()  [unwired: 1 in, 5 out]
        n142 = Bundle By Name(cluster=w415, "Operação"=enum."save - custom") -> (w417:cluster{"Operação":T2, "data":variant})
        n143 = Enqueue Element(queue=w418, element=w417, error in (no error)=w419) -> (queue out=w421:refnum<queue>, error out=w420:errorcluster)  [unwired: 1 in, 1 out]
      }
      event "Salvar - opções": Value Change {
        # "Habilita/desabilita as formas de \"salvar\""
        n144 = event-data() -> ()  [unwired: 1 in, 5 out]
        n145 = property on="Salvar - opções" class="Enum (strict)"(error in=w430) -> (error out=w429:errorcluster, "Value"=w433:enum16{"Default", "Custom"})  [unwired: 1 in, 1 out]
        n146 = case shown="\"Default\", Default" w433 {
          tunnel: w432 -> [w436 w439]
          tunnel: [w436 w439] -> w431
          tunnel: w429 -> [w434 w438]
          tunnel: [w434 w438] -> w426
          tunnel: [T5."Disabled and Grayed Out" ("Disabled") T5."Enabled" ("Disabled")] -> w425
          frame "Default", Default {
          }
          frame "Custom" {
          }
        }
        n147 = property on="Salvar" class="Path"(error in=w426, "DisabledEnum"=w425) -> (error out=w427:errorcluster)  [unwired: 1 in, 1 out]
      }
      event "Salvar - opções 2": Value Change {
        # "Habilita/desabilita as formas de \"salvar\""
        n148 = event-data() -> ()  [unwired: 1 in, 5 out]
        n149 = property on="Salvar - opções 2" class="Enum (strict)"(error in=w446) -> (error out=w445:errorcluster, "Value"=w444:enum16{"Default", "Custom"})  [unwired: 1 in, 1 out]
        n150 = case shown="\"Default\", Default" w444 {
          tunnel: w449 -> [w452 w455]
          tunnel: [w452 w455] -> w448
          tunnel: w445 -> [w450 w454]
          tunnel: [w450 w454] -> w442
          tunnel: [T5."Disabled and Grayed Out" ("Disabled") T5."Enabled" ("Disabled")] -> w443
          frame "Default", Default {
          }
          frame "Custom" {
          }
        }
        n151 = property on="Salvar 2" class="Path"(error in=w442, "DisabledEnum"=w443) -> (error out=w441:errorcluster)  [unwired: 1 in, 1 out]
      }
      event "load1": Value Change {
        w456 = T2[] [enum."load1", enum."display -edit"] items=["update", "write", "stop", "save", "load1", "load2", "add", "sub", "delete", "display", "display -edit", "conc", "HW in", "HW out start", "HW out stop", "initialize", "canal out", "canal in", "save - custom"]
        # "Carrega uma onda para o canal 1"
        n152 = event-data() -> ()  [unwired: 1 in, 5 out]
        n153 = for {
          tunnel: w456 -> [w468] mode=indexing
          tunnel: w457 -> [w464]
          shift-right: [w466] -> w459
          shift-left: w462 -> [w470]
          shift-right: [w467] -> w460
          shift-left: w461 -> [w469]
          n154 = Bundle By Name(cluster=w464, "Operação"=w468) -> (w465:cluster{"Operação":T2, "data":variant})
          n155 = Enqueue Element(queue=w469, element=w465, error in (no error)=w470) -> (queue out=w467:refnum<queue>, error out=w466:errorcluster)  [unwired: 1 in, 1 out]
        }
      }
      event "load2": Value Change {
        w471 = T2[] [enum."load2", enum."display -edit"] items=["update", "write", "stop", "save", "load1", "load2", "add", "sub", "delete", "display", "display -edit", "conc", "HW in", "HW out start", "HW out stop", "initialize", "canal out", "canal in", "save - custom"]
        # "Carrega uma onda para o canal 2"
        n156 = event-data() -> ()  [unwired: 1 in, 5 out]
        n157 = for {
          tunnel: w472 -> [w480]
          shift-right: [w482] -> w474
          shift-left: w477 -> [w485]
          shift-right: [w483] -> w475
          shift-left: w476 -> [w484]
          tunnel: w471 -> [w479] mode=indexing
          n158 = Bundle By Name(cluster=w480, "Operação"=w479) -> (w481:cluster{"Operação":T2, "data":variant})
          n159 = Enqueue Element(queue=w484, element=w481, error in (no error)=w485) -> (queue out=w483:refnum<queue>, error out=w482:errorcluster)  [unwired: 1 in, 1 out]
        }
      }
      event "Add": Value Change {
        w486 = T2[] [enum."add", enum."display -edit"] items=["update", "write", "stop", "save", "load1", "load2", "add", "sub", "delete", "display", "display -edit", "conc", "HW in", "HW out start", "HW out stop", "initialize", "canal out", "canal in", "save - custom"]
        # "Adição"
        n160 = event-data() -> ()  [unwired: 1 in, 5 out]
        n161 = for {
          tunnel: w486 -> [w498] mode=indexing
          tunnel: w487 -> [w494]
          shift-right: [w496] -> w489
          shift-left: w492 -> [w500]
          shift-right: [w497] -> w490
          shift-left: w491 -> [w499]
          n162 = Bundle By Name(cluster=w494, "Operação"=w498) -> (w495:cluster{"Operação":T2, "data":variant})
          n163 = Enqueue Element(queue=w499, element=w495, error in (no error)=w500) -> (queue out=w497:refnum<queue>, error out=w496:errorcluster)  [unwired: 1 in, 1 out]
        }
      }
      event "Gerar": Value Change {
        # "Encerrar geração"
        # "Iniciar geração"
        # "Saída do HW"
        n164 = event-data() -> ()  [unwired: 1 in, 5 out]
        n165 = Select(t=enum."HW out start" ("Operação"), s="Gerar", f=enum."HW out stop" ("Operação")) -> (s? t:f=w504:T2)
        n166 = Bundle By Name(cluster=w505, "Operação"=w504) -> (w507:cluster{"Operação":T2, "data":variant})
        n167 = Enqueue Element(queue=w509, element=w507, error in (no error)=w510) -> (queue out=w512:refnum<queue>, error out=w511:errorcluster)  [unwired: 1 in, 1 out]
      }
      event "Adquirir": Value Change {
        # "Entrada do HW"
        n168 = event-data() -> ()  [unwired: 1 in, 5 out]
        n169 = Bundle By Name(cluster=w515, "Operação"=enum."HW in") -> (w513:cluster{"Operação":T2, "data":variant})
        n170 = Enqueue Element(queue=w520, element=w513, error in (no error)=w518) -> (queue out=w516:refnum<queue>, error out=w517:errorcluster)  [unwired: 1 in, 1 out]
      }
      event "Sub": Value Change {
        w522 = T2[] [enum."sub", enum."display -edit"] items=["update", "write", "stop", "save", "load1", "load2", "add", "sub", "delete", "display", "display -edit", "conc", "HW in", "HW out start", "HW out stop", "initialize", "canal out", "canal in", "save - custom"]
        # "Subtração"
        n171 = event-data() -> ()  [unwired: 1 in, 5 out]
        n172 = for {
          tunnel: w522 -> [w534] mode=indexing
          tunnel: w523 -> [w530]
          shift-right: [w532] -> w525
          shift-left: w528 -> [w536]
          shift-right: [w533] -> w526
          shift-left: w527 -> [w535]
          n173 = Bundle By Name(cluster=w530, "Operação"=w534) -> (w531:cluster{"Operação":T2, "data":variant})
          n174 = Enqueue Element(queue=w535, element=w531, error in (no error)=w536) -> (queue out=w533:refnum<queue>, error out=w532:errorcluster)  [unwired: 1 in, 1 out]
        }
      }
      event "Conc": Value Change {
        w537 = T2[] [enum."conc", enum."display -edit"] items=["update", "write", "stop", "save", "load1", "load2", "add", "sub", "delete", "display", "display -edit", "conc", "HW in", "HW out start", "HW out stop", "initialize", "canal out", "canal in", "save - custom"]
        # "Concatena ondas"
        n175 = event-data() -> ()  [unwired: 1 in, 5 out]
        n176 = for {
          tunnel: w538 -> [w546]
          shift-right: [w548] -> w540
          shift-left: w543 -> [w551]
          shift-right: [w549] -> w541
          shift-left: w542 -> [w550]
          tunnel: w537 -> [w545] mode=indexing
          n177 = Bundle By Name(cluster=w546, "Operação"=w545) -> (w547:cluster{"Operação":T2, "data":variant})
          n178 = Enqueue Element(queue=w550, element=w547, error in (no error)=w551) -> (queue out=w549:refnum<queue>, error out=w548:errorcluster)  [unwired: 1 in, 1 out]
        }
      }
      event "delete": Value Change {
        w552 = T2[] [enum."delete", enum."display -edit"] items=["update", "write", "stop", "save", "load1", "load2", "add", "sub", "delete", "display", "display -edit", "conc", "HW in", "HW out start", "HW out stop", "initialize", "canal out", "canal in", "save - custom"]
        # "Deleta trecho da onda"
        n179 = event-data() -> ()  [unwired: 1 in, 5 out]
        n180 = for {
          tunnel: w552 -> [w564] mode=indexing
          tunnel: w553 -> [w560]
          shift-right: [w562] -> w555
          shift-left: w558 -> [w566]
          shift-right: [w563] -> w556
          shift-left: w557 -> [w565]
          n181 = Bundle By Name(cluster=w560, "Operação"=w564) -> (w561:cluster{"Operação":T2, "data":variant})
          n182 = Enqueue Element(queue=w565, element=w561, error in (no error)=w566) -> (queue out=w563:refnum<queue>, error out=w562:errorcluster)  [unwired: 1 in, 1 out]
        }
      }
      event "Escala X": Value Change {
        # "Escala X do display de edição"
        n183 = event-data() -> ()  [unwired: 1 in, 5 out]
        n184 = property on="Sinal 2" class="WFGraph (strict)"("XScale.Maximum"="Escala X", "XScale.Minimum"=0.0 ("X Scale.Range:Minimum")) -> ()  [unwired: 2 in, 2 out]
      }
      event "Ch1", "Ch2": Value Change {
        # "Liga/desliga os canais do display de edição"
        n185 = event-data() -> ()  [unwired: 1 in, 5 out]
        n186 = Bundle By Name(cluster=w573, "Operação"=enum."display -edit") -> (w575:cluster{"Operação":T2, "data":variant})
        n187 = Enqueue Element(queue=w578, element=w575, error in (no error)=w577) -> (queue out=w580:refnum<queue>, error out=w579:errorcluster)  [unwired: 1 in, 1 out]
      }
      event "Canal out": Value Change {
        # "Liga/desliga os canais do display de edição"
        n188 = event-data() -> ()  [unwired: 1 in, 5 out]
        n189 = Bundle By Name(cluster=w582, "Operação"=enum."canal out") -> (w584:cluster{"Operação":T2, "data":variant})
        n190 = Enqueue Element(queue=w587, element=w584, error in (no error)=w586) -> (queue out=w589:refnum<queue>, error out=w588:errorcluster)  [unwired: 1 in, 1 out]
      }
      event "Input": Value Change {
        # "Liga/desliga os canais do display de edição"
        n191 = event-data() -> ()  [unwired: 1 in, 5 out]
        n192 = Bundle By Name(cluster=w591, "Operação"=enum."canal in") -> (w593:cluster{"Operação":T2, "data":variant})
        n193 = Enqueue Element(queue=w596, element=w593, error in (no error)=w595) -> (queue out=w598:refnum<queue>, error out=w597:errorcluster)  [unwired: 1 in, 1 out]
      }
      event "stop": Value Change {
        w600 = T2[] [enum."display -edit", enum."stop", enum."display", enum."HW out stop"] items=["update", "write", "stop", "save", "load1", "load2", "add", "sub", "delete", "display", "display -edit", "conc", "HW in", "HW out start", "HW out stop", "initialize", "canal out", "canal in", "save - custom"]
        # "Encerra as operações"
        n194 = event-data() -> ()  [unwired: 1 in, 3 out]
        n195 = for {
          tunnel: w600 -> [w612] mode=indexing
          tunnel: w601 -> [w608]
          shift-right: [w611] -> w604
          shift-left: w606 -> [w614]
          shift-right: [w610] -> w603
          shift-left: w605 -> [w613]
          n196 = Bundle By Name(cluster=w608, "Operação"=w612) -> (w609:cluster{"Operação":T2, "data":variant})
          n197 = Enqueue Element At Opposite End(queue=w614, element=w609, error in (no error)=w613) -> (queue out=w611:refnum<queue>, error out=w610:errorcluster)  [unwired: 1 in, 1 out]
        }
      }
    }
  }
  n198 = Merge Errors(w2, w1) -> (w3:errorcluster)
  n199 = Release Queue(queue=w14, error in (no error)=w3) -> (error out=w13:errorcluster)  [unwired: 1 in, 2 out]
  n200 = call <vilib>:"Simple Error Handler.vi"("error in (no error)"=w13) -> ()  [unwired: 4 in, 5 out]
